vi "Delete All Properties.vi"   [LabVIEW 2015]
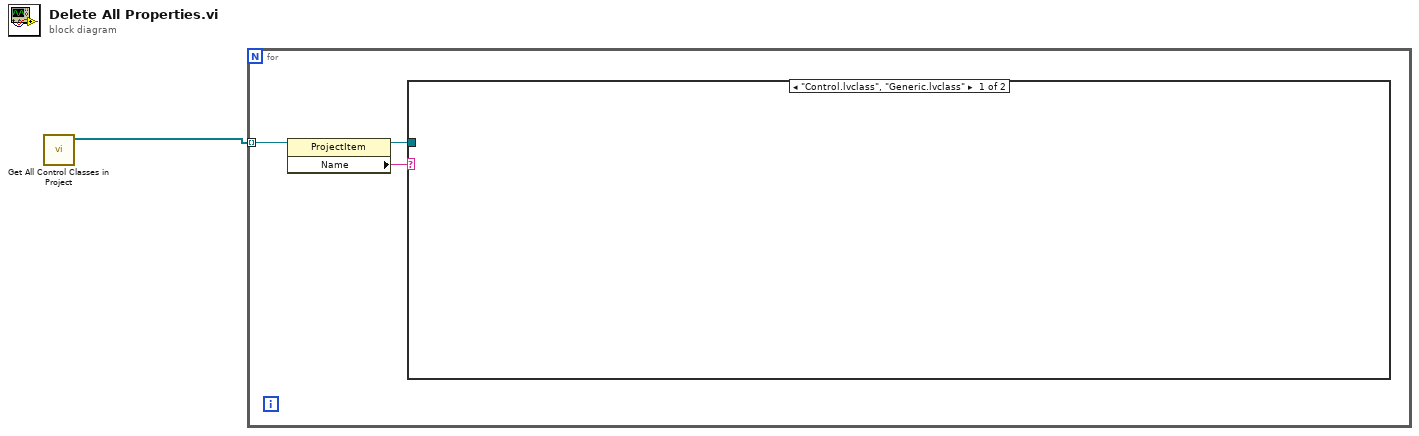
[diagram p0: block diagram]
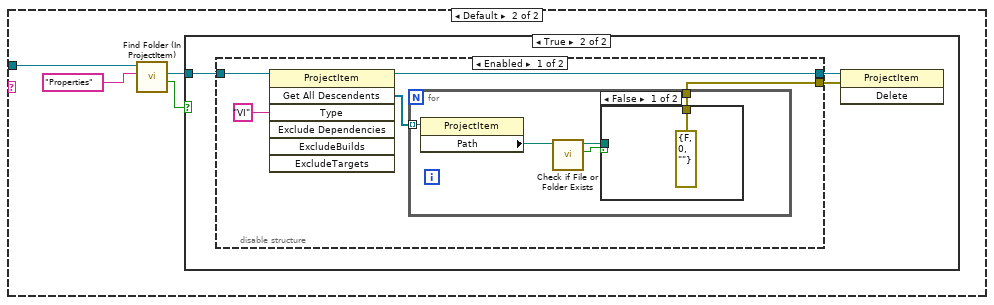
[diagram p2: hidden frame]
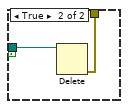
[diagram p4: hidden frame]
diagram:
  n1 = call "Get All Control Classes in Project.vi"() -> ("All Control Classes"=w1:refnum<vi>[])  [unwired: 11 in]
  n2 = for {
    tunnel: w1 -> [w4] mode=indexing
    n3 = property class="ProjectItem"(reference=w4) -> (reference out=w2:refnum<vi>, "Name"=w3:string)  [unwired: 1 in, 1 out]
    n4 = case shown="\"Control.lvclass\", \"Generic.lvclass\"" w3 {
      tunnel: w2 -> [_ w8]
      frame "Control.lvclass", "Generic.lvclass" {
      }
      frame Default {
        n5 = call "Find Folder (In ProjectItem).vi"("Folder Name"="Properties", "ProjectItem in"=w8) -> ("Found?"=w5:bool, "Folder Refnum"=w6:refnum<vi>)  [unwired: 7 in, 1 out]
        n6 = case shown="True" w5 {
          tunnel: w6 -> [_ w11]
          frame False {
          }
          frame True {
            n7 = disable-structure shown="Enabled" {
              disable-tunnel: w11 -> [w16 w25]
              disable-tunnel: [w15 w25] -> w10
              disable-tunnel: [w14 _] -> w9
              frame Enabled {
                n8 = invoke class="ProjectItem" method="Get All Descendents"(reference=w16, "Type"="VI") -> (reference out=w15:refnum<vi>, "All Descendents"=w13:refnum<vi>[])  [unwired: 5 in, 5 out]
                n9 = for {
                  tunnel: w13 -> [w21] mode=indexing
                  tunnel: [w20] -> w14
                  n10 = property class="ProjectItem"(reference=w21) -> ("Path"=w19:path)  [unwired: 1 in, 2 out]
                  n11 = call <vilib>:"Check if File or Folder Exists.vi"("path"=w19) -> ("file or folder exists?"=w17:bool, "dup path"=w18:path)  [unwired: 8 in, 1 out]
                  n12 = case shown="False" w17 {
                    tunnel: [errorcluster {"status"=FALSE, "code"=0, "source"=""} ("error out") w24] -> w20
                    tunnel: w18 -> [_ w23]
                    frame False {
                    }
                    frame True {
                      n13 = Delete(path (use dialog)=w23) -> (error out=w24:errorcluster)  [unwired: 4 in, 2 out]
                    }
                  }
                }
              }
              frame Disabled {
              }
            }
            n14 = invoke class="ProjectItem" method="Delete"(reference=w10, error in=w9) -> ()  [unwired: 1 in, 3 out]
          }
        }
      }
    }
  }
